vi "BooleanCtlTest.vi"() -> ()   [LabVIEW 2016]
uses:
  APIs/Get/GetVI/GetVIByPath.vi
  APIs/Stimulus/VI/OpenVIFrontPanel.vi
  APIs/Stimulus/VI/RunVI.vi
  APIs/Stimulus/VI/MakeVIFrontMost.vi
  APIs/Stimulus/KeyBoardSimulation/ValueSignalLatchBooleanString.vi
  APIs/Assert/AssertControlValue/Equal.vi
  Drona.lvlib
  APIs/Get/GetVI/GetVI.lvlib
  <vilib>/addons/_JKI Toolkits/Caraya/classes/Test/Test.lvclass
  apis/Assert/AssertControlValue/AssertControlValue.lvlib
  apis/Stimulus/KeyBoardSimulation/KeyboardSimulation.lvlib
  apis/Stimulus/VI/VI.lvlib
panel:
  out "error out":errorcluster
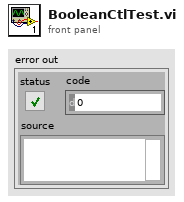
[diagram p1: front panel]
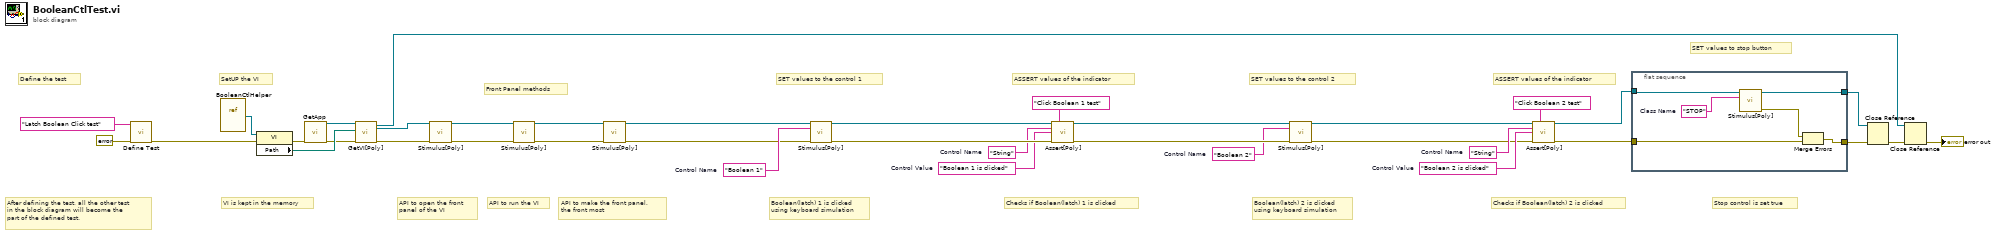
[diagram p0: block diagram]
diagram:
  w23 = "String"  # Control Name
  w21 = "Boolean 2 is clicked"  # Control Value
  w10 = "Boolean 2"  # Control Name
  w24 = "String"  # Control Name
  w28 = "Boolean 1 is clicked"  # Control Value
  w26 = "Boolean 1"  # Control Name
  # "API to make the front panel, \nthe front most"
  # "Front Panel methods"
  # "Stop control is set true"
  # "SET values to stop button"
  # "API to open the front\npanel of the VI"
  # "Checks if Boolean(latch) 2 is clicked"
  # "ASSERT values of the indicator"
  # "Boolean(latch) 2 is clicked\nusing keyboard simulation"
  # "SET values to the control 2"
  # "Checks if Boolean(latch) 1 is clicked"
  # "ASSERT values of the indicator"
  # "Boolean(latch) 1 is clicked\nusing keyboard simulation"
  # "API to run the VI"
  # "SET values to the control 1"
  # "VI is kept in the memory"
  # "SetUP the VI"
  # "After defining the test, all the other test\nin the block diagram will become the \npart of the defined test."
  # "Define the test"
  n1 = call <vilib>:"Define Test.vi"("error in (no error)"=errorcluster {"status"=FALSE, "code"=0, "source"=""}, "Label (VI Title)"="Latch Boolean Click test") -> ("error out"=w32:errorcluster)  [unwired: 9 in]
  n2 = vi-ref "BooleanCtlHelper.vi"() -> (w25:refnum<vi>)
  n3 = property on="Property Node" class="VI"(reference=w25, error in=w32) -> (error out=w36:errorcluster, "Path"=w35:path)  [unwired: 1 out]
  n4 = call "GetApp.vi"("error in (no error)"=w36) -> ("Application Ref"=w37:refnum<vi>, "error out"=w34:errorcluster)  [unwired: 13 in]
  n5 = call-poly "GetVI[Poly].vi"("Application Ref in"=w37, "VI Path"=w35, "error in (no error)"=w34) -> ("Application Ref out"=w1:refnum<vi>, "VI Reference"=w14:refnum<vi>, "error out"=w15:errorcluster)  [unwired: 10 in]
  n6 = call-poly "Stimulus[Poly].vi"("VI Reference In"=w14, "error in"=w15) -> ("VI Reference Out"=w12:refnum<vi>, "error out"=w13:errorcluster)  [unwired: 12 in]
  n7 = call-poly "Stimulus[Poly].vi"("VI Reference In"=w12, "error in"=w13) -> ("VI Reference Out"=w4:refnum<vi>, "error out"=w6:errorcluster)  [unwired: 12 in]
  n8 = call-poly "Stimulus[Poly].vi"("VI Reference In"=w4, "error in"=w6) -> ("VI Reference Out"=w3:refnum<vi>, "error out"=w5:errorcluster)  [unwired: 12 in]
  n9 = call-poly "Stimulus[Poly].vi"("VI Reference In"=w3, "Control Path"=w26, "error in"=w5) -> ("VI Reference Out"=w29:refnum<vi>, "error out"=w30:errorcluster)  [unwired: 11 in]
  n10 = call-poly "Assert[Poly].vi"("VI Reference In"=w29, "Label"="Click Boolean 1 test" ("Label (VI Title)"), "Control Path"=w24, "Control Value"=w28, "Error In"=w30) -> ("VI Reference Out"=w9:refnum<vi>, "Error Out"=w11:errorcluster)  [unwired: 9 in]
  n11 = call-poly "Stimulus[Poly].vi"("VI Reference In"=w9, "Control Path"=w10, "error in"=w11) -> ("VI Reference Out"=w7:refnum<vi>, "error out"=w8:errorcluster)  [unwired: 11 in]
  n12 = call-poly "Assert[Poly].vi"("VI Reference In"=w7, "Label"="Click Boolean 2 test" ("Label (VI Title)"), "Control Path"=w23, "Control Value"=w21, "Error In"=w8) -> ("VI Reference Out"=w17:refnum<vi>, "Error Out"=w19:errorcluster)  [unwired: 9 in]
  n13 = flat-sequence {
    tunnel: [w43] -> w18
    tunnel: [w39] -> w16
    tunnel: w17 -> [w41]
    tunnel: w19 -> [w42]
    frame #0 {
      w40 = "STOP"  # Class Name
      n14 = call-poly "Stimulus[Poly].vi"("VI Reference In"=w41, "Control Path"=w40) -> ("VI Reference Out"=w39:refnum<vi>, "error out"=w38:errorcluster)  [unwired: 12 in]
      n15 = Merge Errors(w38, w42) -> (w43:errorcluster)
    }
  }
  n16 = Close Reference(reference=w16, error in (no error)=w18) -> (error out=w20:errorcluster)
  n17 = Close Reference(reference=w1, error in (no error)=w20) -> (error out=→"error out":errorcluster)
